vi "Master Reference Not Closed--error.vi"() -> (0 "error out":errorcluster)   [LabVIEW 2020, in "My Cloneable Module.lvlib"]
doc: "Outputs an error cluster containing a custom error code indicating the module cannot be run as singleton because it was previously run as cloneable and the master reference is still open.\n_____\nBased on Delacor QMH Project Template 5.1.0.87."
uses:
  My Cloneable Module.lvlib
  <vilib>/Utility/error.llb/Error Cluster From Error Code.vi
  <vilib>/ErrorRing/Error Ring.xnode
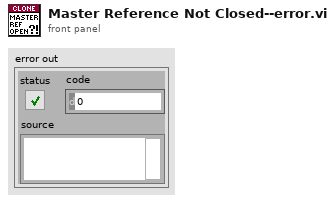
[diagram p1: front panel]
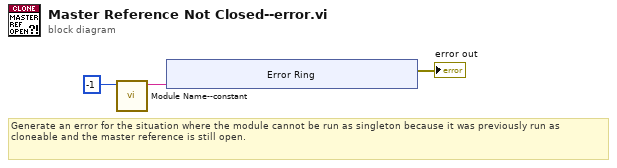
[diagram p0: block diagram]
diagram:
  # "Generate an error for the situation where the module cannot be run as singleton because it was previously run as cloneable and the master reference is still open."
  n1 = call "Module Name--constant.vi"("Module ID"=-1) -> ("Module Name"=w1:string)  [unwired: 10 in]
  n2 = xnode "Error Ring"("parameter 0"=w1) -> ("error out"=→"error out":errorcluster)
